vi "test_ccd_acquireImage.vi"(8 "error in":errorcluster, 11 "CCD in":refnum<class "CCD.lvclass">) -> (0 "error out":errorcluster, 3 "CCD out":refnum<class "CCD.lvclass">)   [LabVIEW 2023, in "horiba.test.lvlib"]
uses:
  horiba.test.lvlib
  Classes/CCD/CCD.lvclass
  C:/Projects/Horiba/horiba-labview-sdk/Source/Classes/GenericDevice/GenericDevice.lvclass
  f7563d15-716f-4b44-beb1-7a38c7aa8869.vi
  <vilib>/addons/_JKI Toolkits/Caraya/classes/Assert/Assert Equal Value_Variant.vi
  <vilib>/addons/_JKI Toolkits/Caraya/classes/Test/Test.lvclass
  <vilib>/addons/_JKI Toolkits/Caraya/classes/Assert/Assert.lvclass
  <userlib>/_OpenG.lib/lvdata/lvdata.llb/openg_variant.lvlib
  <vilib>/JDP Science/JDP Science Common Utilities/JDP Utility.lvlib
panel:
  # "Connector Pane"
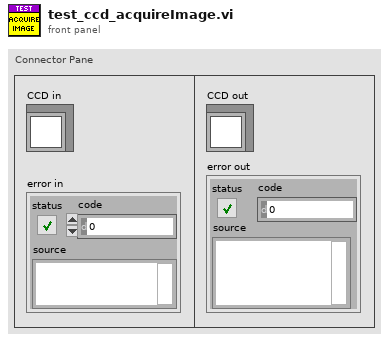
[diagram p1: front panel]
types:
  T1 = cluster{"ROI-index":i32, "xOrigin":i32, "yOrigin":i32, "xSize":i32, "ySize":i32, "xBin":i32, "yBin":i32}
  T2 = cluster{"acqIndex":i32, "roiIndex":i32, "xBinning":i32, "xOrigin":i32, "xSize":i32, "yBinning":i32, "yOrigin":i32, "ySize":i32, "xAxis":dbl[], "number of columns":i32, "matrix":i32}
  T3 = typedef "horiba.lvlib/CCD.lvclass/ccdAcquisitionData.ctl" = cluster{"acqIndex":i32, "ROIs":T4[], "timestamp":string}
  T4 = typedef "horiba.lvlib/CCD.lvclass/imageAcqData.ctl" = cluster{"roiMetaData":T5, "xAxis":dbl[], "yData":dbl[][]}
  T5 = typedef "horiba.lvlib/CCD.lvclass/roiMetaData.ctl" = cluster{"roiIndex":i32, "xBinning":i32, "xOrigin":i32, "xSize":i32, "yBinning":i32, "yOrigin":i32, "ySize":i32}
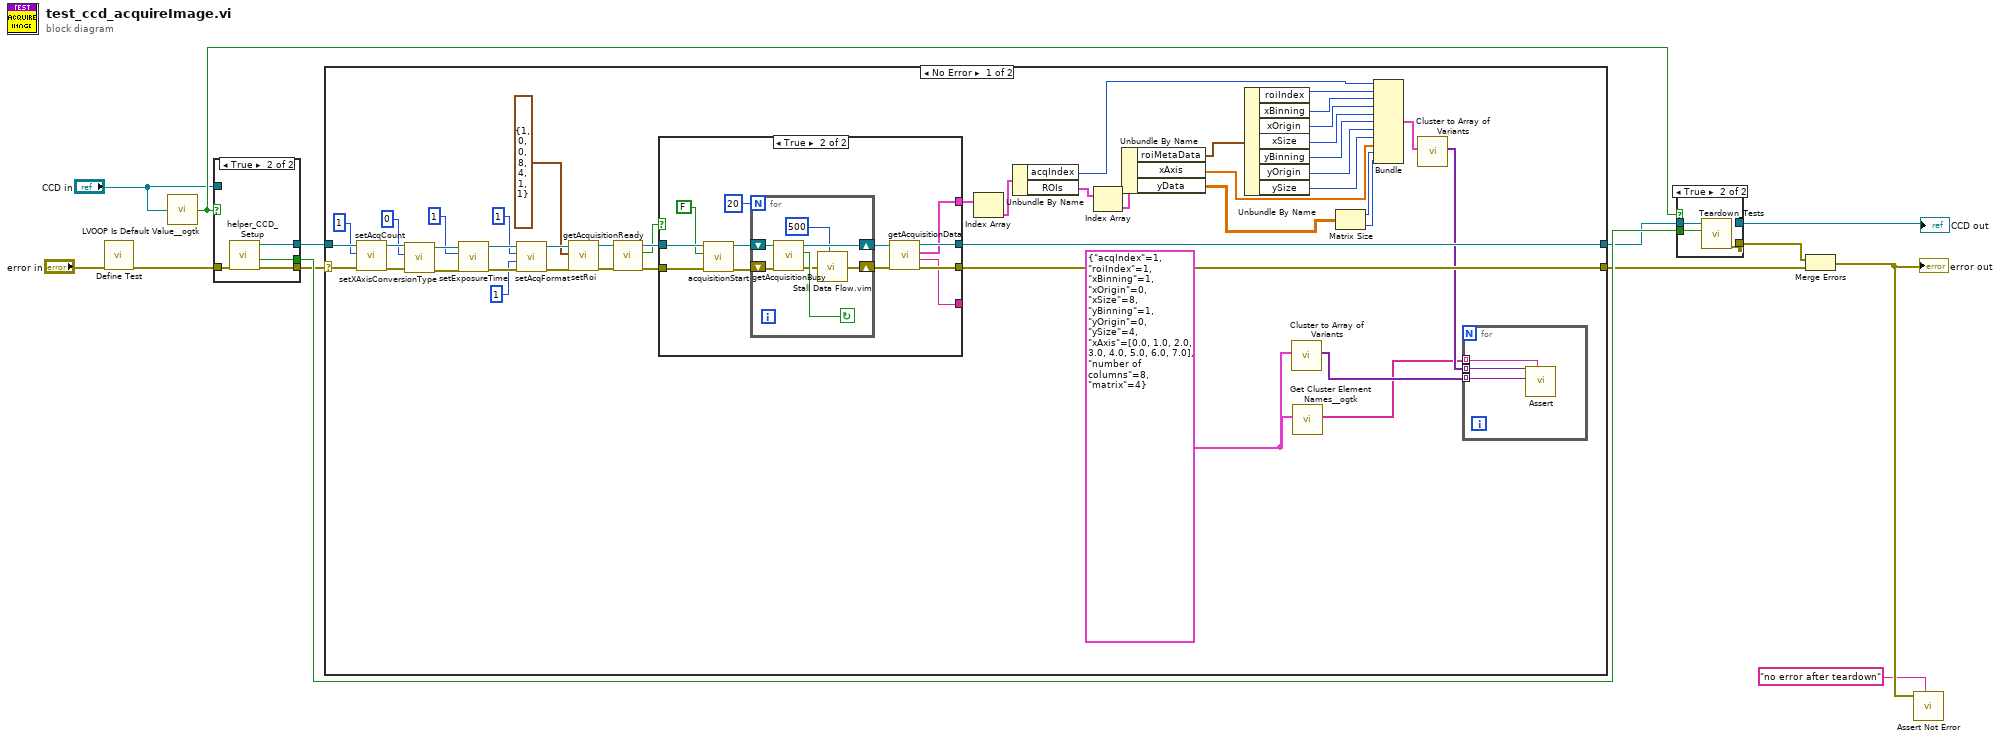
[diagram p0: block diagram]
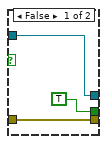
[diagram p3: hidden frame]
diagram:
  n1 = call <vilib>:"Define Test.vi"("error in (no error)"="error in") -> ("error out"=w8:errorcluster)  [unwired: 9 in, 1 out]
  n2 = call <userlib>:"LVOOP Is Default Value__ogtk.vi"("Object"="CCD in") -> ("Is Default Value?"=w9:bool)
  n3 = case shown="True" w9 {
    tunnel: w8 -> [w15 w20]
    tunnel: [w15 w19] -> w4
    tunnel: [w16 w18] -> w6
    tunnel: [TRUE ("Module Was Already Running?") w17] -> w10
    tunnel: "CCD in" -> [w16 _]
    frame False {
    }
    frame True {
      n4 = call "helper_CCD_Setup.vi"("error in"=w20) -> ("error out"=w19:errorcluster, "Module Was Already Running?"=w17:bool, "CCD out"=w18:refnum<class "CCD.lvclass">)  [unwired: 7 in, 1 out]
    }
  }
  n5 = case shown="No Error" w4 {
    selector: w4 -> [w65 w91]
    tunnel: [w44 w90] -> w5
    tunnel: w6 -> [w64 w90]
    tunnel: [w45 w91] -> w3
    frame No Error {
      w28 = T2 {"acqIndex"=1, "roiIndex"=1, "xBinning"=1, "xOrigin"=0, "xSize"=8, "yBinning"=1, "yOrigin"=0, "ySize"=4, "xAxis"=[0.0, 1.0, 2.0, 3.0, 4.0, 5.0, 6.0, 7.0], "number of columns"=8, "matrix"=4} ("output cluster")
      n6 = call "setAcqCount.vi"("error in (no error)"=w65, "count"=1, "CCD in"=w64) -> ("error out"=w62:errorcluster, "CCD out"=w61:refnum<class "CCD.lvclass">)  [unwired: 5 in, 2 out]
      n7 = call "setXAxisConversionType.vi"("error in (no error)"=w62, "type"=0, "CCD in"=w61) -> ("error out"=w59:errorcluster, "CCD out"=w58:refnum<class "CCD.lvclass">)  [unwired: 5 in, 2 out]
      n8 = call "setExposureTime.vi"("error in (no error)"=w59, "exposure time [ms] or [us]"=1, "CCD in"=w58) -> ("error out"=w56:errorcluster, "CCD out"=w55:refnum<class "CCD.lvclass">)  [unwired: 5 in, 2 out]
      n9 = call "setAcqFormat.vi"("error in (no error)"=w56, "format"=1, "number of ROIs"=1, "CCD in"=w55) -> ("error out"=w52:errorcluster, "CCD out"=w51:refnum<class "CCD.lvclass">)  [unwired: 4 in, 2 out]
      n10 = call "setRoi.vi"("error in (no error)"=w52, "roiConfig"=T1 {"ROI-index"=1, "xOrigin"=0, "yOrigin"=0, "xSize"=8, "ySize"=4, "xBin"=1, "yBin"=1}, "CCD in"=w51) -> ("error out"=w49:errorcluster, "CCD out"=w48:refnum<class "CCD.lvclass">)  [unwired: 5 in, 2 out]
      n11 = call "getAcquisitionReady.vi"("error in (no error)"=w49, "CCD in"=w48) -> ("error out"=w47:errorcluster, "ready"=w43:bool, "CCD out"=w46:refnum<class "CCD.lvclass">)  [unwired: 7 in]
      n12 = case shown="True" w43 {
        tunnel: w47 -> [w69 w82]
        tunnel: w46 -> [w70 w81]
        tunnel: [w69 w75] -> w45
        tunnel: [w70 w73] -> w44
        tunnel: [_ w72] -> _
        tunnel: [_ w71] -> w42
        frame False {
        }
        frame True {
          n13 = call "acquisitionStart.vi"("error in (no error)"=w82, "openShutter"=FALSE, "CCD in"=w81) -> ("error out"=w77:errorcluster, "CCD out"=w76:refnum<class "CCD.lvclass">)  [unwired: 5 in, 2 out]
          n14 = for {
            N: 20 -> [_]
            shift-right: [w85] -> w78
            shift-left: w77 -> [w88]
            shift-right: [w84] -> w74
            shift-left: w76 -> [w89]
            stop <- w87 continue-if-true
            n15 = call "getAcquisitionBusy.vi"("error in (no error)"=w88, "CCD in"=w89) -> ("error out"=w86:errorcluster, "isBusy"=w87:bool, "CCD out"=w84:refnum<class "CCD.lvclass">)  [unwired: 7 in]
            n16 = call "Stall Data Flow.vim"("value in"=w86, "milliseconds to wait"=u32 500) -> ("value out"=w85:errorcluster)  [unwired: 1 out]
          }
          n17 = call "getAcquisitionData.vi"("error in (no error)"=w78, "CCD in"=w74) -> ("error out"=w75:errorcluster, "results-JSON string"=w72:string, "ccdAcquisitions"=w71:T3[], "CCD out"=w73:refnum<class "CCD.lvclass">)  [unwired: 6 in]
        }
      }
      n18 = Index Array(array=w42) -> (element=w41:T3)  [unwired: 1 in]
      n19 = Unbundle By Name(w41) -> ("acqIndex"=w29:i32, "ROIs"=w40:T4[])
      n20 = Index Array(array=w40) -> (element=w39:T4)  [unwired: 1 in]
      n21 = Unbundle By Name(w39) -> ("roiMetaData"=w23:T5, "xAxis"=w22:dbl[], "yData"=w21:dbl[][])
      n22 = Unbundle By Name(w23) -> ("roiIndex"=w38:i32, "xBinning"=w37:i32, "xOrigin"=w36:i32, "xSize"=w35:i32, "yBinning"=w34:i32, "yOrigin"=w33:i32, "ySize"=w32:i32)
      n23 = call <vilib>:"Cluster to Array of Variants.vi"("Cluster"=w28) -> ("Array of Cluster Elements"=w25:variant[])  [unwired: 10 in]
      n24 = call <userlib>:"Get Cluster Element Names__ogtk.vi"("Cluster"=w28) -> ("Element Names"=w24:string[])  [unwired: 9 in, 1 out]
      n25 = Matrix Size(0:w21) -> (1:w31:i32, 2:w30:i32)
      n26 = Bundle("acqIndex"=w29, "roiIndex"=w38, "xBinning"=w37, "xOrigin"=w36, "xSize"=w35, "yBinning"=w34, "yOrigin"=w33, "ySize"=w32, "xAxis"=w22, "number of columns"=w31, "matrix"=w30) -> (w27:T2)  [unwired: 1 in]
      n27 = call <vilib>:"Cluster to Array of Variants.vi"("Cluster"=w27) -> ("Array of Cluster Elements"=w26:variant[])  [unwired: 10 in]
      n28 = for {
        tunnel: w26 -> [w68] mode=indexing
        tunnel: w25 -> [w67] mode=indexing
        tunnel: w24 -> [w66] mode=indexing
        n29 = call-poly <vilib>:"Assert.vi"("Label"=w66, "Y"=w67, "X"=w68) -> ()  [unwired: 7 in, 2 out]
      }
    }
    frame Error {
    }
  }
  n30 = case shown="True" w9 {
    tunnel: w5 -> [w92 w95]
    tunnel: [_ w94] -> w7
    tunnel: w10 -> [_ w93]
    tunnel: [w92 _] -> w1
    frame False {
    }
    frame True {
      n31 = call "Teardown_Tests.vi"("Module Was Already Running?"=w93, "horiba.lvlib:GenericDevice"=w95) -> ("error out"=w94:errorcluster)  [unwired: 8 in, 1 out]
    }
  }
  "CCD out" <- w1
  n32 = Merge Errors(w7, w3) -> (w12:errorcluster)
  "error out" <- w12
  n33 = call <vilib>:"Assert Not Error.vi"("Label"="no error after teardown", "Not Error?"=w12) -> ()  [unwired: 8 in, 2 out]
